vi "Launch_Server.vi"(7 "port":u16=6379, 8 "error in":errorcluster, 10 "working directory":path, 11 "host":string="localhost") -> (0 "error out":errorcluster, 2 "Server Alive ?":bool)   [LabVIEW 2023]
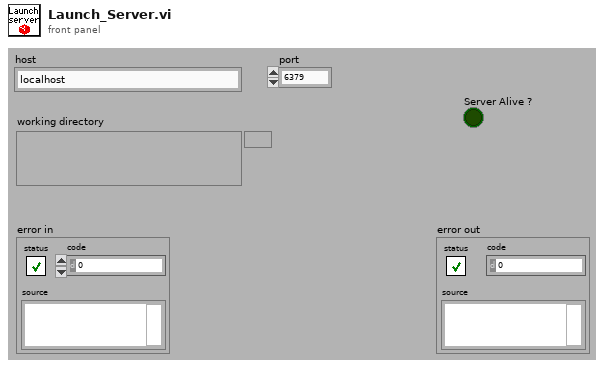
[diagram p1: front panel]
types:
  T1 = enum16{"None", "Error", "Status", "Nil", "Integer", "String", "Multibulk"}
  T2 = cluster{"integer":i64, "string":string, "multibulk":variant[]}
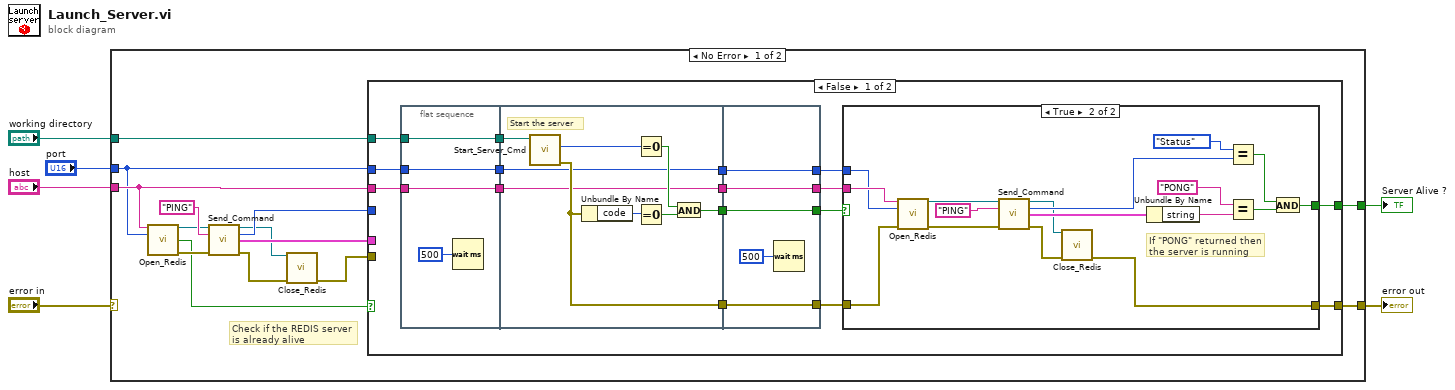
[diagram p0: block diagram]
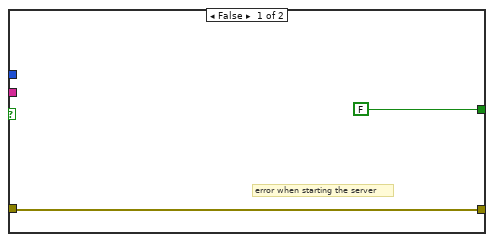
[diagram p2: hidden frame]
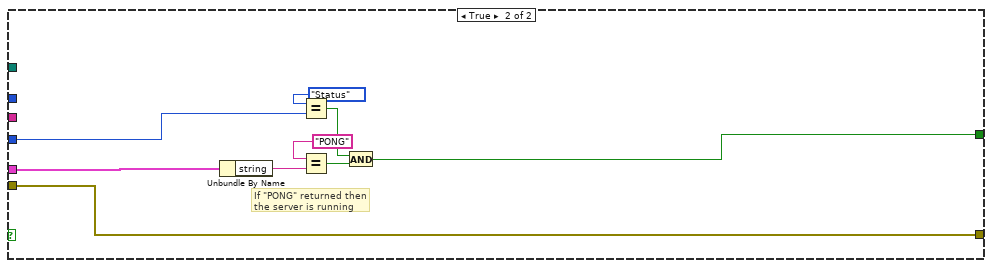
[diagram p3: hidden frame]
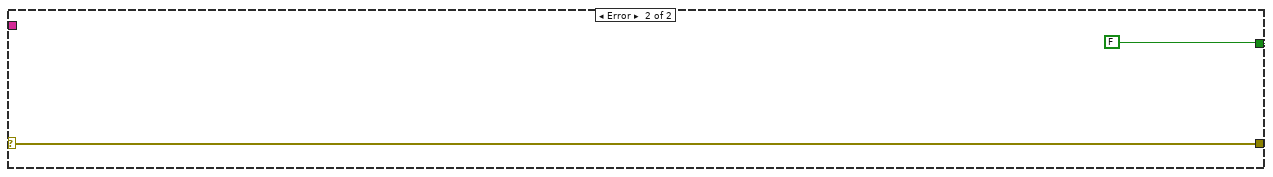
[diagram p4: hidden frame]
diagram:
  n1 = case shown="No Error" "error in" {
    selector: "error in" -> [_ w84]
    tunnel: "host" -> [w14 _]
    tunnel: [w17 w84] -> w4
    tunnel: "working directory" -> [w16 _]
    tunnel: [w15 FALSE] -> w2
    tunnel: "port" -> [w7 _]
    frame No Error {
      # "Check if the REDIS server\nis already alive"
      n2 = call "Open_Redis.vi"("Host"=w14, "Port"=w7) -> ("TCP session out"=w13:refnum<k5>, "Connection ok ?"=w11:bool, "error out"=w12:errorcluster)  [unwired: 11 in]
      n3 = call "Send_Command.vi"("TCP session in"=w13, "command"="PING", "error in"=w12) -> ("TCP session out"=w10:refnum<k5>, "type"=w18:T1, "reply"=w19:T2, "error out"=w9:errorcluster)  [unwired: 8 in, 1 out]
      n4 = call "Close_Redis.vi"("TCP session in"=w10, "error in"=w9) -> ("error out"=w8:errorcluster)  [unwired: 10 in, 3 out]
      n5 = case shown="False" w11 {
        tunnel: w19 -> [_ w80]
        tunnel: w18 -> [_ w82]
        tunnel: [w32 w74] -> w17
        tunnel: w16 -> [w36 _]
        tunnel: [w34 w75] -> w15
        tunnel: w14 -> [w24 _]
        tunnel: w7 -> [w28 _]
        tunnel: w8 -> [_ w74]
        frame False {
          n6 = flat-sequence {
            tunnel: w36 -> [w40]
            tunnel: [w40] -> w31
            tunnel: w28 -> [w39]
            tunnel: [w39] -> w27
            tunnel: w24 -> [w38]
            tunnel: [w38] -> w23
            tunnel: w31 -> [w45]
            tunnel: [w44] -> w30
            tunnel: [w43] -> w29
            tunnel: w27 -> [w42]
            tunnel: [w42] -> w26
            tunnel: w23 -> [w41]
            tunnel: [w41] -> w22
            tunnel: [w53] -> w33
            tunnel: [w54] -> w35
            tunnel: w30 -> [w54]
            tunnel: w29 -> [w53]
            tunnel: w26 -> [w52]
            tunnel: [w52] -> w25
            tunnel: w22 -> [w51]
            tunnel: [w51] -> w21
            frame #0 {
              n7 = Wait (ms)(milliseconds to wait=u32 500) -> ()  [unwired: 1 out]
            }
            frame #1 {
              # "Start the server"
              n8 = call "Start_Server_Cmd.vi"("working directory"=w45) -> ("error out"=w43:errorcluster, "return code"=w46:i32)  [unwired: 9 in]
              n9 = Unbundle By Name(w43) -> ("code"=w47:i32)
              n10 = Equal To 0?(x=w46) -> (x = 0?=w49:bool)
              n11 = Equal To 0?(x=w47) -> (x = 0?=w48:bool)
              n12 = And(x=w49, y=w48) -> (x .and. y?=w44:bool)
            }
            frame #2 {
              n13 = Wait (ms)(milliseconds to wait=u32 500) -> ()  [unwired: 1 out]
            }
          }
          n14 = case shown="True" w35 {
            tunnel: w21 -> [_ w63]
            tunnel: w25 -> [_ w62]
            tunnel: [FALSE w65] -> w34
            tunnel: w33 -> [w55 w64]
            tunnel: [w55 w57] -> w32
            frame False {
              # "error when starting the server"
            }
            frame True {
              # "If \"PONG\" returned then\nthe server is running"
              n15 = call "Open_Redis.vi"("Host"=w63, "Port"=w62, "error in"=w64) -> ("TCP session out"=w61:refnum<k5>, "error out"=w60:errorcluster)  [unwired: 10 in, 1 out]
              n16 = call "Send_Command.vi"("TCP session in"=w61, "command"="PING", "error in"=w60) -> ("TCP session out"=w58:refnum<k5>, "type"=w73:T1, "reply"=w72:T2, "error out"=w59:errorcluster)  [unwired: 8 in, 1 out]
              n17 = call "Close_Redis.vi"("TCP session in"=w58, "error in"=w59) -> ("error out"=w57:errorcluster)  [unwired: 10 in, 3 out]
              n18 = Unbundle By Name(w72) -> ("string"=w70:string)
              n19 = Equal?(x=T1."Status" ("type"), y=w73) -> (x = y?=w67:bool)
              n20 = Equal?(x="PONG", y=w70) -> (x = y?=w68:bool)
              n21 = And(x=w67, y=w68) -> (x .and. y?=w65:bool)
            }
          }
        }
        frame True {
          # "If \"PONG\" returned then\nthe server is running"
          n22 = Unbundle By Name(w80) -> ("string"=w79:string)
          n23 = Equal?(x=T1."Status" ("type"), y=w82) -> (x = y?=w76:bool)
          n24 = Equal?(x="PONG", y=w79) -> (x = y?=w77:bool)
          n25 = And(x=w76, y=w77) -> (x .and. y?=w75:bool)
        }
      }
    }
    frame Error {
    }
  }
  "error out" <- w4
  "Server Alive ?" <- w2
